vi "camera-build-pixel-array.vi"(1 "size":dbl, 2 "step":dbl, 3 "start":dbl) -> (0 "construction":dbl[](array[numeric]))   [LabVIEW 2015]
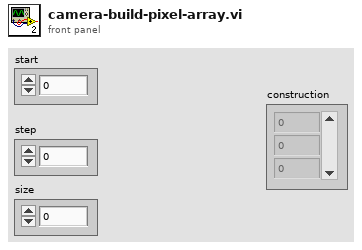
[diagram p1: front panel]
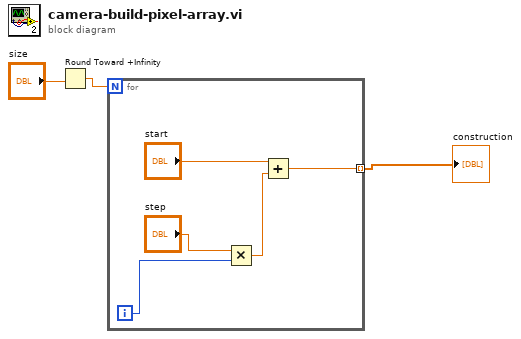
[diagram p0: block diagram]
diagram:
  n1 = Round Toward +Infinity(x="size") -> (ceil(x): smallest int >= x=w1:dbl)
  n2 = for {
    N: w1 -> [_]
    tunnel: [w4] -> w3 mode=indexing
    i -> [w8]
    n3 = Multiply(x="step", y=w8) -> (x*y=w5:dbl)
    n4 = Add(x="start", y=w5) -> (x+y=w4:dbl)
  }
  "construction" <- w3
